vi "UHR-Fleezers Control (host) - 11.9b.vi"() -> ()   [LabVIEW 2014] (continued)
  # "Fl. Up"
  # "Bead sep"
  # "Trap Display:"
  # "APD Display:"
  # "Trap Manipulation"
  # "Data Saving"
  # "DAQ"
  # "Bead Calibration"
  # "Tether screen"
  # "Bottom Pump (#1)"
  # "Central Sample Channels"
  # "Top Pump (#3)"
  # "Rate param is ul/h\nVolume param is ul"
  # "Chemyx Pump 2"
  # "Units: \n1 = ml/m\n2 = ml/h\n3 = ul/m\n4 = ul/h"
  # "X"
  # "Y"
  # "Oscillate Set 1 freq. (debugging)"
  # "BD 1"
  # "BD 2"
  # "AOD Raster Scan"
  # "Approx. trap separations"
  # "X"
  # "Y"
  # "FPGA\nreading"
  # "DMA\ntransfer"
  # "APD Gates"
  # "APD 2"
  # "APD 1"
  # "X"
  # "2D"
  # "Y"
  # "1D"
  # "Green Laser Interlacing"
  # "Green FB Measurement"
  # "Digital Gate"
  # "Current Analog Control"
  # "Total AI Rates (NOT rates/trap)"
  # "(Samples/trap x Trap Sets)"
  # "(Samples/channel x\n8 if averaging (8 channels)\n4 if no averaging)"
  # "Trap 1"
  # "Trap 2"
  # "Flour./Trap 3"
  # "External Video Window"
  # "MCL Position Debugging"
  # "Temporary Control Storage\n(these used to be somewhere else, still want to keep them)"
  # "Y"
  # "X"
  # "Trap Position Difference Limits"
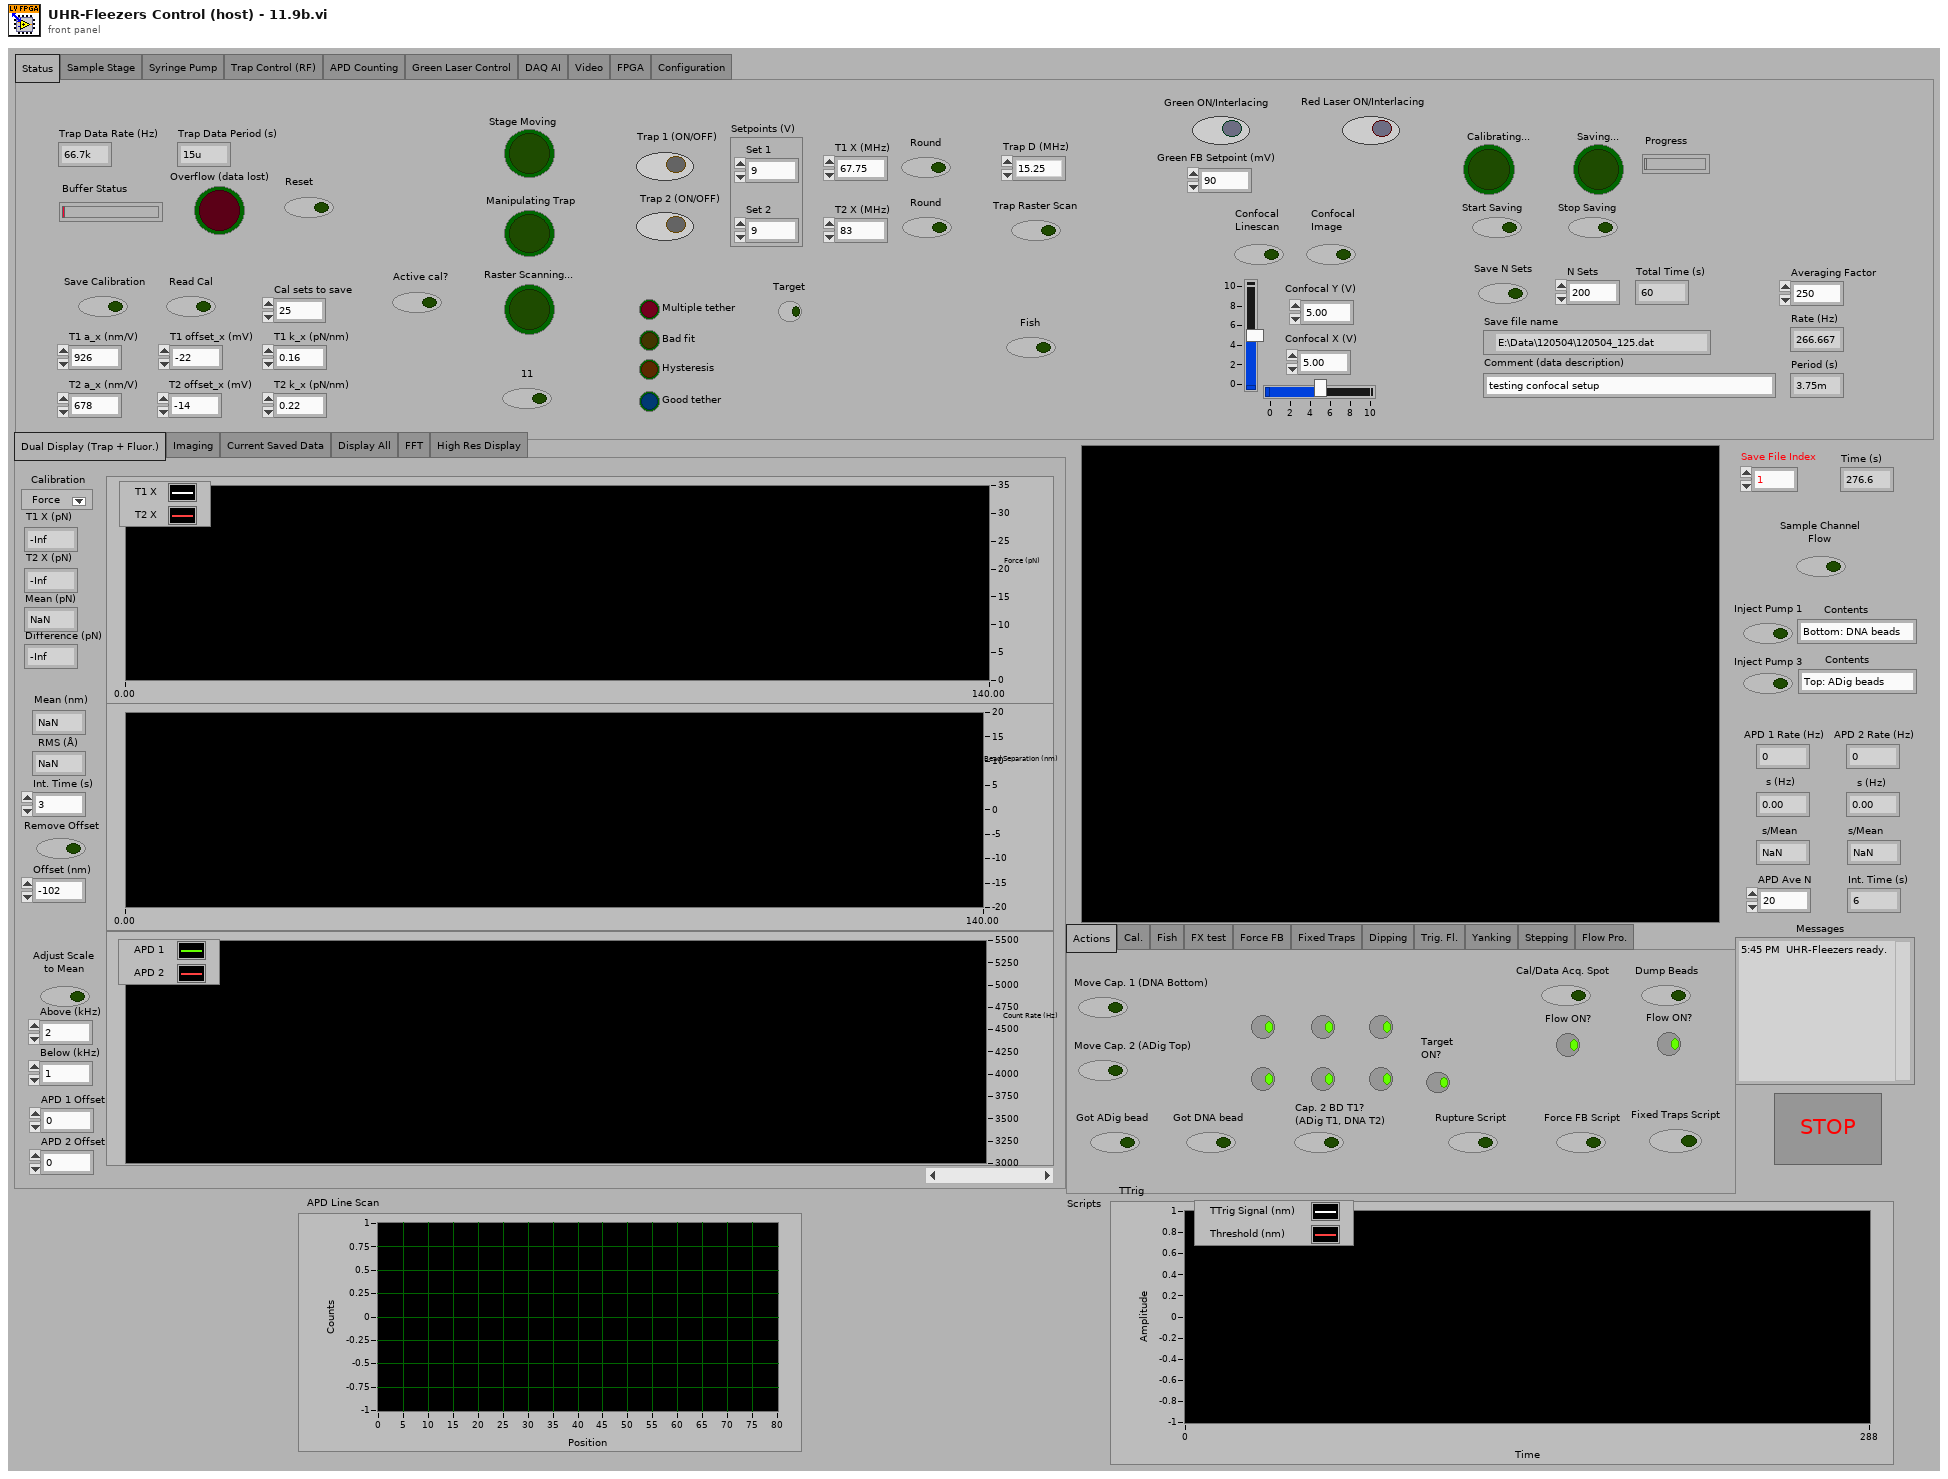
[diagram p1: front panel]
types:
  T1 = enum32{"Actions", "Cal.", "Fish", "FX test", "Force FB", "Fixed Traps", "Dipping", "Trig. Fl.", "Yanking", "Stepping", "Flow Pro."}
  T2 = typedef "IMAQ Image.ctl" = refnum<image>
  T3 = enum32{"Dual Display (Trap + Fluor.)", "Imaging", "Current Saved Data", "Display All", "FFT", "High Res Display"}
  T4 = enum32{"Status", "Sample Stage", "Syringe Pump", "Trap Control (RF)", "APD Counting", "Green Laser Control", "DAQ AI", "Video", "FPGA", "Configuration"}
  T5 = cluster{"Pump 1":cluster{"Diameter (mm)":dbl, "Units":dbl, "Volume":dbl, "Rate":dbl}, "Pump 2":cluster{"Diameter (mm)":dbl, "Units":dbl, "Volume":dbl, "Rate":dbl}, "Pump 3":cluster{"Diameter (mm)":dbl, "Units":dbl, "Volume":dbl, "Rate":dbl}}
  T6 = enum32{"IR Laser Interlacing (Direct RF Board Control Method)", "AOD Raster Scan", "Feedback on Trap Intensity", "Feedback on Trap Position"}
  T7 = typedef "LVPoint32TypeDef.ctl" = cluster{"Horizontal":i32, "Vertical":i32}
  T8 = cluster{"Scan Range AOD (nm) 2":dbl, "Step Size AOD (nm) 2":dbl, "Scan Speed AOD (nm/s) 2":dbl, "Number of scans (AOD) 2":u16, "Label":string}[]
  T9 = cluster{"Set 1":cluster{"proportional gain (Kc)":i16, "integral gain (Kc*Ts/Ti)":i16, "derivative gain (Kc*Td/Ts)":i16}, "Set 2":cluster{"proportional gain (Kc)":i16, "integral gain (Kc*Ts/Ti)":i16, "derivative gain (Kc*Td/Ts)":i16}}
  T10 = cluster{"Trap 1":fxp<+/-,16,1>, "Trap 2":fxp<+/-,16,1>}
  T11 = cluster{"proportional gain (Kc)":fxp<+/-,16,8>, "integral gain (Kc*Ts/Ti)":fxp<+/-,16,8>, "derivative gain (Kc*Td/Ts)":fxp<+/-,16,8>}
  T12 = cluster{"output high":fxp<+/-,64,32>, "output low":fxp<+/-,64,32>}
  T13 = cluster{"Set 1":fxp<+/-,16,1>, "Set 2":fxp<+/-,16,1>}
  T14 = cluster{"proportional gain (Kc)":i16, "integral gain (Kc*Ts/Ti)":i16, "derivative gain (Kc*Td/Ts)":i16}
  T15 = cluster{"Set 1":bool, "Set 2":bool, "Set 3":bool}
  T16 = typedef "LVMinMaxIncTypeDef.ctl" = cluster{"Minimum":dbl, "Maximum":dbl, "Increment":dbl}
  T17 = typedef "Image Type" = u32
  T18 = typedef "nirio_resource_hc.ctl" = tag
  T19 = typedef "openfpgaref.8.6.ctl" = refnum<k20>
  T20 = cluster{"New Image":T2, "New Image":T2, "New Image":T2, "New Image":T2}
  T21 = typedef "XDNodeRunTimeDep.lvlib/timing_clust.ctl" = cluster{"Expected End [f-1]":u64, "Actual End [f-1]":u64, "Finished Late? [f-1]":bool, "Expected End [i-1]":u64, "Actual End [i-1]":u64, "Finished Late? [i-1]":bool, "Expected Start [i]":u64, "Actual Start [i]":u64, "Expected Start [f]":u64, "Actual Start [f]":u64, "Source Name":string, "Structure Name":string, "Period":i64, "Deadline":i64, "Offset":i64, "Start":i64, "Priority":i32, "Timeout":i32, "Mode":T22, "Wakeup Reason":T23, "Error":errorcluster, "Source Type":string, "Secondary Source Type":string, "Global End Time":u64, "Global Start Time":u64, "Frame Duration":u64, "Iteration Duration":u64, "Assigned CPU":i32, "I/O Scan Engine Mode":u32}
  T22 = typedef "XDNodeRunTimeDep.lvlib/nitl_modes.ctl" = enum32{"No Change", "Process missed periods, maintain original phase", "Discard missed periods, maintain original phase", "Process missed periods, ignore original phase", "Discard missed periods, ignore original phase"}
  T23 = typedef "XDNodeRunTimeDep.lvlib/wakeup.ctl" = enum32{"Normal", "Aborted", "Asynchronous wakeup", "Timing source error", "Timed loop error", "Timeout"}
  T24 = enum16{"big-endian, network order", "native, host order", "little-endian"}
  T25 = enum16{"open", "replace", "create", "open or create", "replace or create", "replace or create with confirmation"}
  T26 = cluster{"Scan Range AOD (nm) 2":dbl, "Step Size AOD (nm) 2":dbl, "Scan Speed AOD (nm/s) 2":dbl, "Number of scans (AOD) 2":u16, "Label":string}
  T27 = cluster{"[0]":dbl, "[1]":dbl, "[2]":dbl, "[3]":dbl, "[4]":dbl, "[5]":dbl}
  T28 = cluster{"Diameter (mm)":dbl, "Units":dbl, "Volume":dbl, "Rate":dbl}
  T29 = enum16{"Actions", "Cal.", "Fish", "FX test", "Force FB", "Fixed Traps", "Dipping", "Trig. Fl.", "Yanking", "Stepping", "Flow Pro."}
  T30 = cluster{"Left":i32, "Top":i32, "Width":u32, "Height":u32}
  T31 = cluster{cluster{"Left":i32, "Top":i32, "Width":u32, "Height":u32}}[]
  T32 = enum32{"setting", "request", "request control", "info", "statistics", "system settings", "I/O sub system", "HRT control", "camera descriptions", "device specific data", "event sub system settings", "event sub system results", "image memory manager"}
  T33 = typedef "AviRefnum.ctl" = refnum<k1>
  T34 = typedef "imagedata.ctl" = cluster{"image type":i32, "image depth":i32, "image":u8[], "mask":u8[], "colors":u32[], "Rectangle":cluster{"left":i16, "top":i16, "right":i16, "bottom":i16}}
  T35 = enum32{"Normal Display", "Dual Display (APD)", "FFT", "High Res Display"}
  T36 = cluster{"Origin Pixel":cluster{"X":sgl, "Y":sgl}, "Angle Relative to Horizontal (deg)":sgl, "Axis Reference":u32}
  T37 = typedef "Simple Grid Descriptor" = cluster{"X Step":sgl, "Y Step":sgl, "Unit":T38}
  T38 = typedef "Image Unit" = enum32{"Undefined", "Angström", "Micrometer", "Millimeter", "Centimeter", "Meter", "Kilometer", "Microinch", "Inch", "Feet", "Nautical miles", "Standard miles", "Steps"}
  T39 = cluster{"averaging mode":u16, "weighting mode":u16, "number of averages":u32}
  T40 = cluster{"dB On (F)":bool, "unwrap phase (F)":bool, "convert to degree (F)":bool}
  T41 = cluster{string, string, string, string, string, string, string, string}
  T42 = cluster{string, string, string, string, string, string, string, string, string, string, string, string}
  T43 = cluster{string, string, string, string, string, string, string, string, string, string, string, string, string}
  T44 = cluster{string, string, string, string, string, string, string, string, string, string, string, string, string, string}
  T45 = cluster{"BD 1 Frequency 1 (MHz)":dbl, "BD 1 Frequency 2 (MHz)":dbl}
  T46 = cluster{"f0":dbl, "df":dbl, "magnitude":dbl[]}[][]
  T47 = cluster{"Green FB Ch 0":i16, "Green FB Ch 1":i16, "Green FB Ch 2":i16}
  T48 = cluster{"Green FB Ch 0":dbl, "Green FB Ch 1":dbl, "Green FB Ch 2":dbl}
diagram:
  w17 = 0.0 ("Total Volume\nFlowed P1 (uL)")
  w29 = u16 20 items=["1.0"=10, "1.5"=15, "2.0"=20] ("stop bits (10: 1 bit)")
  w32 = u16 20 items=["1.0"=10, "1.5"=15, "2.0"=20] ("stop bits (10: 1 bit)")
  w89 = u16 20 items=["1.0"=10, "1.5"=15, "2.0"=20] ("stop bits (10: 1 bit)")
  w96 = T17 2 items=["Grayscale (U8)", "Grayscale (I16)", "Grayscale (SGL)", "Complex (CSG)", "RGB (U32)", "HSL (U32)", "RGB (U64)", "Grayscale (U16)"] ("Image Type")
  w158 = cluster{"output high":i16, "output low":i16} {"output high"=3000, "output low"=0} ("FB output range 1")
  w229 = 10.0 ("y")
  w228 = 32767.0 ("y")
  w244 = 6.0  # clock mult.
  w245 = 49152000.0  # TCXO frequ.
  # "Bottom 1 Harvard"
  # "Top 3 Harvard"
  # "Center Harvard"
  # "Bottom 1 Harvard"
  # "Top 3 Harvard"
  # "Center Harvard"
  n1 = Build Array("DIO count 1 (ticks)", "DIO count 2 (ticks)", "DIO count 3 (ticks)") -> (w145:u32[])
  n2 = local read "AO1"() -> (w223:dbl)
  n3 = local read "AO2"() -> (w222:dbl)
  n4 = local read "Scan Increment (MHz)"() -> (w240:dbl)
  n5 = local read "Continuous MCL Scanning"() -> (w210:bool)
  n6 = local read "Fast Scan Dir"() -> (w209:bool)
  n7 = local read "Number of scans (MCL)"() -> (w211:u64)
  n8 = property on="AI Count (ticks)" class="DigNum (strict)"("Val(Sgnl)"="AI Count (ticks)") -> ()  [unwired: 2 in, 2 out]
  n9 = Multiply(x=w223, y=w228) -> (x*y=w225:dbl)
  n10 = Multiply(x=w222, y=w228) -> (x*y=w227:dbl)
  n11 = Divide(x=w225, y=w229) -> (x/y=w224:dbl)
  n12 = Divide(x=w227, y=w229) -> (x/y=w226:dbl)
  n13 = To Word Integer(number=w224) -> (16bit integer=w221:i16)
  n14 = To Word Integer(number=w226) -> (16bit integer=w220:i16)
  n15 = Not(x=w209) -> (.not. x?=w204:bool)
  n16 = local read "Cycles/step (MCL)"() -> (w212:u64)
  n17 = Multiply(x=w240, y=1000.0) -> (x*y=w247:dbl)
  n18 = local read "Scan steps (MCL)"() -> (w213:u64)
  n19 = local write "Trap Pos FIFO Timeout"(u16 0 ("Trap Pos FIFO Timeout")) -> ()
  n20 = local read "Desired Scan Incr (V)"() -> (w215:dbl)
  n21 = Scale By Power Of 2(n=48, x=w247) -> (x*2^n=w248:dbl)
  n22 = Multiply(x=w245, y=w244) -> (x*y=w243:dbl)
  n23 = Divide(x=w248, y=w243) -> (x/y=w242:dbl)
  n24 = local read "Setpoints (V)"() -> (w259:cluster{"Set 1":dbl, "Set 2":dbl})
  n25 = To Quad Integer(1:w242) -> (0:w239:i64)
  n26 = Divide(x=40000000.0, y="AI Count (ticks)") -> (x/y=w200:dbl)
  n27 = Multiply(x=w215, y=32767.0) -> (x*y=w217:dbl)
  n28 = local read "Number Interlace Sets"() -> (w138:u8)
  n29 = Split 1D Array(array=w145, index=w138) -> (first subarray=w147:u32[])  [unwired: 1 out]
  n30 = Add Array Elements(numeric array=w147) -> (sum=w146:u32)
  n31 = local read "# Samples/channel"() -> (w232:u32)
  n32 = local read "Number of F/B Scans (AOD)"() -> (w233:u16)
  n33 = local read "Not-Interlacing Set"() -> (w137:enum32{"Set 1", "Set 2", "Set 3"})
  n34 = To Unsigned Byte Integer(number=w137) -> (unsigned 8bit integer=w143:u8)
  n35 = Index Array(array=w145, index=w143) -> (element=w144:u32)
  n36 = local read "Feedback On/Off"() -> (w262:cluster{"Set 1":bool, "Set 2":bool})
  n37 = local read "PID Gains"() -> (w254:T9)
  n38 = local read "Scan steps (AOD)"() -> (w238:u64)
  n39 = local read "All FB On/Off"() -> (w263:bool)
  n40 = local read "Cycles/step (AOD)"() -> (w237:u64)
  n41 = local write "AI rate (Hz)"(w200) -> ()
  n42 = Divide(x=w217, y=10.0) -> (x/y=w216:dbl)
  n43 = Multiply(x=w238, y=w237) -> (x*y=w236:u64)
  n44 = Multiply(x=3276.7, y=w259) -> (x*y=w258:cluster{"Set 1":dbl, "Set 2":dbl})
  n45 = To Word Integer(number=w216) -> (16bit integer=w214:i16)
  n46 = xnode "Open FPGA VI Reference"("resource name"=T18 "RIO1") -> ("FPGA VI Reference Out"=w15:T19, "error out"=w13:errorcluster)  [unwired: 1 in]
  n47 = Multiply(x=w236, y=u64 2) -> (x*y=w234:u64)
  n48 = local read "Sets to FIFO (Traps)"() -> (w266:T15)
  n49 = Divide(x=w200, y="FPGA Ave.") -> (x/y=w201:dbl)
  n50 = To Word Integer(number=w258) -> (16bit integer=w257:cluster{"Set 1":i16, "Set 2":i16})
  n51 = Unbundle By Name(w254) -> ("Set 1"=w253:T14, "Set 2"=w252:T14)
  n52 = Multiply(x=w234, y=w233) -> (x*y=w231:u64)
  n53 = local write "Ave. Rate (Hz)"(w201) -> ()
  n54 = Divide(x=w231, y=w232) -> (x/y=w230:dbl)
  n55 = Unbundle By Name(w257) -> ("Set 1"=w256:i16, "Set 2"=w255:i16)
  n56 = local read "2D or 1D Scan"() -> (w159:bool)
  n57 = local write "Data points/scans"(w231) -> ()
  n58 = local read "Scan BD"() -> (w249:bool)
  n59 = And(x=w262, y=w263) -> (x .and. y?=w261:cluster{"Set 1":bool, "Set 2":bool})
  n60 = local write "Data points/scan (f/b)"(w234) -> ()
  n61 = Reciprocal(x=w201) -> (1/x=w202:dbl)
  n62 = local read "N Acq Sets (Traps + Fl.)"() -> (w193:i16)
  n63 = local write "N sets should be saved"(w230) -> ()
  n64 = xnode "Invoke Method"("FPGA VI Reference In"=w15, "error in"=w13) -> ("FPGA VI Reference Out"=w157:T19, "error out"=w167:errorcluster)
  n65 = Unbundle By Name(w261) -> ("Set 1"=w265:bool, "Set 2"=w264:bool)
  n66 = local read "Interlace"() -> (w139:bool)
  n67 = Select(t=w146, s=w139, f=w144) -> (s? t:f=w136:u32)
  n68 = local write "Update Count (MCL)"(w136) -> ()
  n69 = local write "Total Counts (ticks)"(w136) -> ()
  n70 = local write "Ave. Period (s)"(w202) -> ()
  n71 = property on="2D or 1D Scan" class="Bool (strict)"("Val(Sgnl)"=w159) -> ()  [unwired: 2 in, 2 out]
  n72 = local read "GI Frequency, OFF count"() -> (w61:u32)
  n73 = local read "GI Frequency, ON count"() -> (w52:u32)
  n74 = local read "APD Gate OFF Count"() -> (w58:u32)
  n75 = local read "APD Gate ON Count"() -> (w54:u32)
  n76 = xnode "Read/Write Control"("FPGA VI Reference In"=w156, "error in"=w167, "ai count"="AI Count (ticks)", "Interlace ON/OFF"=w139, "Number Interlace Cycles"=w138, "AI1 Sets to FIFO"=w266, "FB On/Off Set 1"=w265, "FB On/Off Set 2"=w264, "Interlace Off Parameters"=w137, "FB Setpoint Set 1"=w256, "FB Setpoint Set 2"=w255, "FB Gains Set 1"=w253, "FB Gains Set 2"=w252, "FB output range 1"=w158, "FB output range 2"=w158, "Cycles per step"=w237, "Scan BD"=w249, "Number of scans"=w233, "Scan steps"=w238, "Scan freq.  increment"=w239, "AO1"=w221, "AO2"=w220, "Scan freq.  increment (MCL)"=w214, "Scan steps (MCL)"=w213, "Cycles per step (MCL)"=w212, "Number of scans (MCL)"=w211, "MCL count"=w136, "Cont. Scan (MCL)"=w210, "MCL Scan Axis"=w204, "1D or 2D Scan?"=w159, "N of AI1 Int Acq Sets"=w193, "Freq or Amp switch first"="Freq or Amp switch first", "Freq switch delay"="Freq switch delay", "Amp switch delay"="Amp switch delay", "Swap F1 and F2"="Swap F1 and F2", "APD to FIFO"=FALSE, "DIO count 1 (ticks)"="DIO count 1 (ticks)", "DIO count 2 (ticks)"="DIO count 2 (ticks)", "DIO count 3 (ticks)"="DIO count 3 (ticks)") -> ("FPGA VI Reference Out"=w65:T19, "error out"=w63:errorcluster)  [unwired: 1 in]
  n77 = local read "On one out of X cycles"() -> (w60:u32)
  n78 = local read "APD Integration Time (s)"() -> (w44:dbl)
  n79 = local read "DMA Update Period (s)"() -> (w43:dbl)
  n80 = Add(x=w54, y=w58) -> (x+y=w56:u32)
  n81 = Add(x=w52, y=w61) -> (x+y=w59:u32)
  n82 = local read "Green ON/Interlacing"() -> (w134:bool)
  n83 = local read "Green laser mode"() -> (w135:enum32{"Laser ON", "Laser OFF", "Interlace"})
  n84 = Multiply(x=w56, y=w60) -> (x*y=w57:u32)
  n85 = Multiply(x=w60, y=w59) -> (x*y=w51:u32)
  n86 = Reciprocal(x=w44) -> (1/x=w41:dbl)
  n87 = Multiply(x=w44, y=40000000.0) -> (x*y=w40:dbl)
  n88 = Divide(x=w43, y=w44) -> (x/y=w46:dbl)
  n89 = Multiply(x="Current When FB OFF (%)", y=655.35) -> (x*y=w122:dbl)
  n90 = local read "Invert APD Gate"() -> (w50:bool)
  n91 = Multiply(x="Green FB Setpoint (mV)", y=3.2767) -> (x*y=w119:dbl)
  n92 = local read "APD Gate"() -> (w49:enum32{"ON", "OFF", "Interlace"})
  n93 = Subtract(x=w57, y=w54) -> (x-y=w55:u32)
  n94 = local write "Green FB Count"(w51) -> ()
  n95 = local write "APD Acq Rate (Hz)"(w41) -> ()
  n96 = To Unsigned Long Integer(number=w40) -> (unsigned 32bit integer=w38:u32)
  n97 = Multiply(x=2.0, y=w46) -> (x*y=w45:dbl)
  n98 = local read "Invert GI"() -> (w131:bool)
  n99 = To Unsigned Word Integer(number=w122) -> (unsigned 16bit integer=w120:u16)
  n100 = Subtract(x=w51, y=w52) -> (x-y=w53:u32)
  n101 = local write "APD Samples/FIFO Acq."(w46) -> ()
  n102 = To Word Integer(number=w119) -> (16bit integer=w117:i16)
  n103 = local write "APD Elements/DMA read"(w45) -> ()
  n104 = case shown="False" w134 {
    tunnel: w135 -> [_ w291]
    tunnel: [enum32{"Laser ON", "Laser OFF", "Interlace"}."Laser OFF" ("Green laser mode") w291] -> w130
    frame False {
    }
    frame True {
    }
  }
  n105 = local write "APD Int. Count"(w38) -> ()
  n106 = Multiply(x="Red current when FB OFF (%)", y=655.35) -> (x*y=w2:dbl)
  n107 = local read "Trap Pos. AI1 X Pre-scale"() -> (w75:u16)
  n108 = local read "Trap Pos FB Monitor\nT1 or T2"() -> (w82:bool)
  n109 = To Unsigned Word Integer(number=w2) -> (unsigned 16bit integer=w1:u16)
  n110 = local read "Trap Pos FB Int Count"() -> (w69:u16)
  n111 = local read "APD 1 AO Mult."() -> (w48:i16)
  n112 = local read "Trap Pos FB Negate Action"() -> (w81:bool)
  n113 = local read "APD 2 AO Mult."() -> (w47:i16)
  n114 = local read "Trap Pos. FB Offset Factor"() -> (w80:i64)
  n115 = local read "Trap Pos. FB Mult Factor"() -> (w79:i64)
  n116 = local read "Differential FB?"() -> (w35:bool)
  n117 = local read "Neg. TTrig FPGA"() -> (w37:bool)
  n118 = local read "Trap Pos. FB Gains"() -> (w77:T11)
  n119 = local read "Trap Pos. FB Range"() -> (w78:T12)
  n120 = xnode "Read/Write Control"("FPGA VI Reference In"=w65, "error in"=w63, "Invert APD Gate"=w50, "APD Gate ON Count"=w54, "APD Gate OFF Count"=w55, "APD Acq Rate Count"=w38, "APD Gate Operating Mode"=w49, "APD 1 AO scale factor"=w48, "APD 2 AO scale factor"=w47, "Green interlace ON count"=w52, "Green interlace OFF count"=w53, "Green interlace ON count 2"=w52, "Green interlace OFF count 2"=w53, "Green FB Count"=w51) -> ("FPGA VI Reference Out"=w64:T19, "error out"=w62:errorcluster)
  n121 = xnode "Read/Write Control"("FPGA VI Reference In"=w64, "error in"=w62, "Invert GI 2"=w131, "Operating Mode 2"=w130, "Green FB Gains"="Green FB Gains", "Green FB Setpoint"=w117, "Green FB On/Off"="Green FB On/Off", "Current Out"=w120, "Green int current ON count adj"="Green int current ON count adj", "Operating Mode"=w130, "Invert GI"=w131, "Trap Pos FB Monitor T1 or T2"=w82, "Trap Pos FB Negate Action"=w81, "Trap Pos. FB Offset Factor"=w80, "Trap Pos. FB Mult Factor"=w79, "Trap Pos. FB Range"=w78, "Trap Pos. FB Gains"=w77, "Force feedback"=FALSE, "AI1 X Scale"=w75, "Trap Pos to FIFO"=TRUE, "Trap Pos FB Int Count"=w69, "TTrig Negate Pos"=w37, "FB Trig Integrate"="FB Trig Integrate", "Diff FB Measurement?"=w35, "Negate Diff?"="Negate Diff?", "RI Current Out"=w1) -> ("FPGA VI Reference Out"=w132:T19, "error out"=w133:errorcluster)
  n122 = xnode "Invoke Method"("FPGA VI Reference In"=w132, "error in"=w133, "Requested Depth"="Trap AI FIFO Depth") -> ("FPGA VI Reference Out"=w85:T19, "error out"=w84:errorcluster)  [unwired: 1 out]
  n123 = xnode "Invoke Method"("FPGA VI Reference In"=w85, "error in"=w84, "Requested Depth"="Trap Position FIFO Depth") -> ("FPGA VI Reference Out"=w71:T19, "error out"=w70:errorcluster)  [unwired: 1 out]
  n124 = flat-sequence {
    tunnel: w157 -> [w296]
    tunnel: [w296] -> w156
    tunnel: [w295] -> w155
    tunnel: [w294] -> w154
    tunnel: [w292] -> w152
    tunnel: [w293] -> w153
    frame #0 {
      w293 = T16 {"Minimum"=0.0, "Maximum"=40.0, "Increment"=1.0} ("Min Max Inc")
      w292 = T16 {"Minimum"=0.0, "Maximum"=50.0, "Increment"=1.0} ("Data Entry Limits")
      w295 = T16 {"Minimum"=60.0, "Maximum"=90.0, "Increment"=1.0} ("Min Max Inc")
      w294 = T16 {"Minimum"=0.0, "Maximum"=50.0, "Increment"=1.0} ("Data Entry Limits")
      n125 = property on="BD 2 Frequency 1 (MHz)" class="DigNum (strict)"("Data Range"=w293) -> ()  [unwired: 2 in, 2 out]
      n126 = property on="BD 2 Frequency 3 (MHz)" class="DigNum (strict)"("Data Range"=w293) -> ()  [unwired: 2 in, 2 out]
      n127 = property on="BD 2 Frequency 2 (MHz)" class="DigNum (strict)"("Data Range"=w293) -> ()  [unwired: 2 in, 2 out]
      n128 = property on="BD 1 Frequency 1 (MHz)" class="DigNum (strict)"("Data Range"=w295) -> ()  [unwired: 2 in, 2 out]
      n129 = property on="BD 1 Frequency 2 (MHz)" class="DigNum (strict)"("Data Range"=w295) -> ()  [unwired: 2 in, 2 out]
      n130 = property on="BD 1 Frequency 3 (MHz)" class="DigNum (strict)"("Data Range"=w295) -> ()  [unwired: 2 in, 2 out]
      n131 = property on="BD 2 Amplitude 1 (%)" class="DigNum (strict)"("Data Range"=w292) -> ()  [unwired: 2 in, 2 out]
      n132 = property on="BD 2 Amplitude 2 (%)" class="DigNum (strict)"("Data Range"=w292) -> ()  [unwired: 2 in, 2 out]
      n133 = property on="BD 2 Amplitude 3 (%)" class="DigNum (strict)"("Data Range"=w292) -> ()  [unwired: 2 in, 2 out]
      n134 = property on="BD 1 Amplitude 3 (%)" class="DigNum (strict)"("Data Range"=w294) -> ()  [unwired: 2 in, 2 out]
      n135 = property on="BD 1 Amplitude 2 (%)" class="DigNum (strict)"("Data Range"=w294) -> ()  [unwired: 2 in, 2 out]
      n136 = property on="BD 1 Amplitude 1 (%)" class="DigNum (strict)"("Data Range"=w294) -> ()  [unwired: 2 in, 2 out]
      "X RF Frequency Limits (MHz)" <- w295
      "X RF Amplitude Limits (%)" <- w294
      "Y RF Amplitude Limits (%)" <- w292
      "Y RF Frequency Limits (MHz)" <- w293
    }
  }
  n137 = xnode "Invoke Method"("FPGA VI Reference In"=w71, "error in"=w70) -> ("FPGA VI Reference Out"=w166:T19, "error out"=w165:errorcluster)  [unwired: 1 in]
  n138 = flat-sequence "Initial FPGA Loop Relative Phase Adjustment" {
    tunnel: "Initial Phase Adjustment (APD 2 Gate)" -> [w299]
    tunnel: "Initial Phase Adjustment (GI) 2" -> [w300]
    tunnel: "Initial Phase Adj. (MCL)" -> [w298]
    tunnel: w165 -> [w301]
    tunnel: w166 -> [w302]
    tunnel: "Initial Phase Adjustment (GI)" -> [w303]
    tunnel: "Initial Phase Adjustment (AI1)" -> [w304]
    tunnel: [w304] -> w12
    tunnel: [w303] -> w11
    tunnel: [w302] -> w10
    tunnel: [w301] -> w9
    tunnel: [w298] -> w8
    tunnel: [w300] -> w7
    tunnel: [w299] -> w6
    tunnel: [w316] -> w175
    tunnel: [w310] -> w171
    tunnel: "Initial Phase Adjustment (APD Acq)" -> [w309]
    tunnel: "Initial Phase Adjustment (APD 1 Gate)" -> [w308]
    tunnel: "Initial Phase Adjustment (Green FB)" -> [w307]
    tunnel: w12 -> [w315]
    tunnel: w11 -> [w314]
    tunnel: w10 -> [w313]
    tunnel: w9 -> [w312]
    tunnel: w8 -> [w311]
    tunnel: w7 -> [w306]
    tunnel: w6 -> [w305]
    tunnel: w175 -> [w318]
    tunnel: [w319] -> w172
    tunnel: w171 -> [w319]
    tunnel: [w318] -> w170
    tunnel: w172 -> [w322]
    tunnel: w170 -> [w321]
    tunnel: [w324] -> w169
    tunnel: [w323] -> w168
    tunnel: [w326] -> w173
    tunnel: [w327] -> w174
    tunnel: w169 -> [w327]
    tunnel: w168 -> [w326]
    frame #0 {
      n139 = Wait (ms)(milliseconds to wait=u32 100) -> ()  [unwired: 1 out]
    }
    frame #1 {
      n140 = xnode "Read/Write Control"("FPGA VI Reference In"=w313, "error in"=w312, "Phase count adjustment"=w315, "Phase count adjustment (GI)"=w314, "Phase count adjustment (MCL)"=w311, "Phase Count Adjustment (APD Acq)"=w309, "Phase count adjustment (APD 1 Gate)"=w308, "Phase count adjustment (APD 2 Gate)"=w305, "Phase count adjustment (Green FB)"=w307, "Phase count adjustment (GI) 2"=w306) -> ("FPGA VI Reference Out"=w310:T19, "error out"=w316:errorcluster)
    }
    frame #2 {
      n141 = Wait (ms)(milliseconds to wait=u32 100) -> ()  [unwired: 1 out]
    }
    frame #3 {
      w320 = TRUE
      n142 = xnode "Read/Write Control"("FPGA VI Reference In"=w322, "error in"=w321, "+ phase"=w320, "+ phase (GI)"=w320, "+ phase (MCL)"=w320, "+ phase (APD Acq)"=w320, "+ phase (APD 1 Gate)"=w320, "+ phase (APD 2 Gate)"=w320, "+ phase (Green FB)"=w320, "+ phase (GI) 2"=w320) -> ("FPGA VI Reference Out"=w323:T19, "error out"=w324:errorcluster)
    }
    frame #4 {
      n143 = Wait (ms)(milliseconds to wait=u32 100) -> ()  [unwired: 1 out]
    }
  }
  n144 = local read "Phase adj. (Green FB)"() -> (w148:i16)
  n145 = local read "Phase adj. (GI) 2"() -> (w123:i16)
  n146 = local read "Phase adjust (MCL)"() -> (w205:i16)
  n147 = local read "Phase adj. (AI1)"() -> (w207:i16)
  n148 = local read "Phase adj. (GI)"() -> (w206:i16)
  n149 = xnode "Read/Write Control"("FPGA VI Reference In"=w173, "error in"=w174, "Phase count adjustment"=w207, "Phase count adjustment (GI)"=w206, "Phase count adjustment (MCL)"=w205, "Phase Count Adjustment (APD Acq)"="Phase Adj. (APD Acq)", "Phase count adjustment (APD 1 Gate)"="Phase Adj. (APD 1 Gate)", "Phase count adjustment (APD 2 Gate)"="Phase Adj. (APD 2 Gate)", "Phase count adjustment (Green FB)"=w148, "Phase count adjustment (GI) 2"=w123) -> ("FPGA VI Reference Out"=w14:T19, "error out"=w182:errorcluster)
  n150 = call "Initialize RF boards - interlace 3.vi"("error in"=w182, "FPGA VI Reference In"=w14) -> ("error out"=w180:errorcluster, "FPGA VI Reference Out"=w181:T19)
  n151 = call "set RF board frequency - interlace.vi"("Board 2 Frequency Limits"=w153, "Board 1 Frequency Limits"=w155, "error in"=w180, "FPGA VI Reference In"=w181, "Board 2 Frequency 3 (MHz)"="BD 2 Frequency 3 (MHz)", "Board 1 Frequency 3 (MHz)"="BD 1 Frequency 3 (MHz)", "Board 2 Frequency 2 (MHz)"="BD 2 Frequency 2 (MHz)", "Board 2 Frequency 1 (MHz)"="BD 2 Frequency 1 (MHz)", "Board 1 Frequency 2 (MHz)"="BD 1 Frequency 2 (MHz)", "Board 1 Frequency 1  (MHz)"="BD 1 Frequency 1 (MHz)") -> ("error out"=w281:errorcluster, "FPGA VI Reference Out"=w282:T19)
  n152 = call "set RF board amplitude - interlace.vi"("Board 2 Amplitude Limits"=w152, "Board 1 Amplitude Limits"=w154, "error in"=w281, "FPGA VI Reference In"=w282, "Board 2 Amplitude 3 (%)"="BD 2 Amplitude 3 (%)", "Board 1 Amplitude 3 (%)"="BD 1 Amplitude 3 (%)", "Board 2 Amplitude 2 (%)"="BD 2 Amplitude 2 (%)", "Board 2 Amplitude 1 (%)"="BD 2 Amplitude 1 (%)", "Board 1 Amplitude 2 (%)"="BD 1 Amplitude 2 (%)", "Board 1 Amplitude 1 (%)"="BD 1 Amplitude 1 (%)") -> ("error out"=w269:errorcluster, "FPGA VI Reference Out"=w270:T19)
  n153 = flat-sequence {
    tunnel: w270 -> [w337]
    tunnel: w269 -> [w336]
    tunnel: [w335] -> w274
    tunnel: [w334] -> w273
    tunnel: [w341] -> w272
    tunnel: w274 -> [w341]
    tunnel: [w340] -> w271
    tunnel: w273 -> [w340]
    tunnel: w272 -> [w350]
    tunnel: w271 -> [w349]
    tunnel: [w348] -> w23
    tunnel: [w347] -> w72
    frame #0 {
      w328 = FALSE ("Retract Pump 3")
      n154 = local read "Trap 1 (ON/OFF)"() -> (w329:bool)
      n155 = xnode "Read/Write Control"("FPGA VI Reference In"=w337, "error in"=w336, "Direct RF Box  Communication"=FALSE) -> ("FPGA VI Reference Out"=w335:T19, "error out"=w334:errorcluster)
      n156 = local write "Saving..."(FALSE ("Saving Data")) -> ()
      n157 = local write "Stop All"(FALSE ("Stop All")) -> ()
      n158 = local write "Retract Pump 1"(w328) -> ()
      n159 = local write "Retract Pump 3"(w328) -> ()
      n160 = local write "Index"(1.0 ("Index")) -> ()
      n161 = property on="Trap 1 ON" class="Bool (strict)"("Value"=w329) -> ()  [unwired: 2 in, 2 out]
      "Manipulating Trap" <- FALSE ("Manipulating Trap")
    }
    frame #1 {
      n162 = local read "Trap 2 (ON/OFF)"() -> (w339:bool)
      n163 = Wait (ms)(milliseconds to wait=u32 10) -> ()  [unwired: 1 out]
      n164 = property on="Trap 2 ON" class="Bool (strict)"("Val(Sgnl)"=w339) -> ()  [unwired: 2 in, 2 out]
    }
    frame #2 {
      n165 = local read "Scan Range (nm)"() -> (w343:dbl)
      n166 = xnode "Read/Write Control"("FPGA VI Reference In"=w350, "error in"=w349, "FPGA Controls  RF Box"=TRUE ("Direct RF Box  Communication")) -> ("FPGA VI Reference Out"=w348:T19, "error out"=w347:errorcluster)
      n167 = call "Update messages.vi"("Message to add"="UHR-Fleezers ready.", "Old message string"="") -> ("New message string"=w346:string)
      n168 = local write "Messages"(w346) -> ()
      n169 = property on="Scan Range (nm)" class="DigNum (strict)"("Val(Sgnl)"=w343) -> ()  [unwired: 2 in, 2 out]
    }
  }
  n170 = Subtract(x="BD 1 Frequency 1 (MHz)", y="BD 1 Frequency 2 (MHz)") -> (x-y=w192:dbl)
  n171 = Subtract(x="BD 2 Frequency 1 (MHz)", y="BD 2 Frequency 2 (MHz)") -> (x-y=w191:dbl)
  n172 = Square(x=w191) -> (x^2=w189:dbl)
  n173 = Square(x=w192) -> (x^2=w190:dbl)
  n174 = Add(x=w190, y=w189) -> (x+y=w188:dbl)
  n175 = Square Root(x=w188) -> (sqrt(x)=w187:dbl)
  n176 = local write "Trap D (MHz)"(w187) -> ()
  n177 = call "IMAQ Create"("Image Name"="APD 1 Image", "Image Type"=w96) -> ("New Image"=w95:T2)  [unwired: 3 in, 1 out]
  n178 = call "IMAQ Create"("Image Name"="APD 2 Image", "Image Type"=w96) -> ("New Image"=w94:T2)  [unwired: 3 in, 1 out]
  n179 = call "IMAQ Create"("Image Name"="Det. X Image", "Image Type"=w96) -> ("New Image"=w93:T2)  [unwired: 3 in, 1 out]
  n180 = call "IMAQ Create"("Image Name"="Det. Y Image", "Image Type"=w96) -> ("New Image"=w92:T2)  [unwired: 3 in, 1 out]
  n181 = Bundle("New Image"=w95, "New Image"=w94, "New Image"=w93, "New Image"=w92) -> (w91:T20)  [unwired: 1 in]
  n182 = call-poly "VISA Configure Serial Port"("VISA resource name"="Bottom  1 Harvard Syringe Pump Serial Port", "baud rate (9600)"=u32 115200, "stop bits (10: 1 bit)"=w29) -> ("VISA resource name out"=w25:refnum<visa-resource-name>, "error out"=w24:errorcluster)  [unwired: 4 in, 7 out]
  n183 = call-poly "VISA Configure Serial Port"("VISA resource name"="Top 3 Harvard Syringe Pump Serial Port", "baud rate (9600)"=u32 115200, "stop bits (10: 1 bit)"=w32) -> ("VISA resource name out"=w27:refnum<visa-resource-name>, "error out"=w26:errorcluster)  [unwired: 4 in, 7 out]
  n184 = call-poly "VISA Configure Serial Port"("VISA resource name"="Sample Chamber Stage Serial Port") -> ("VISA resource name out"=w105:refnum<visa-resource-name>, "error out"=w106:errorcluster)  [unwired: 5 in, 8 out]
  "Stage Control Serial Error" <- w106
  n185 = call-poly "VISA Configure Serial Port"("VISA resource name"="Center Harvard Syringe Pump Serial Port", "baud rate (9600)"=u32 115200, "stop bits (10: 1 bit)"=w89) -> ("VISA resource name out"=w86:refnum<visa-resource-name>, "error out"=w87:errorcluster)  [unwired: 4 in, 7 out]
  n186 = disable-structure shown="Disabled" {
    disable-tunnel: [w353 _] -> w251
    disable-tunnel: w23 -> [w352 _]
    frame Disabled {
      n187 = node-c288() -> (w355:T21)  [unwired: 4 out]
      n188 = timed-loop "Rough control of MCL mirror stage (debugging)" {
        tunnel: w352 -> [w358]
        tunnel: [w357] -> w353
        timing: w355 -> [_]
        timing-out: [_] -> w354
        stop <- w357 stop-if-true
        n189 = node-c288() -> ()  [unwired: 2 out]
        n190 = case shown="1" "MCL Mode" {
          tunnel: w358 -> [_ w361 w408]
          frame 0, Default {
          }
          frame 1 {
            n191 = node-c288() -> (w363:T21)  [unwired: 4 out]
            n192 = timed-loop "Oscillate MCL mirror" {
              timing: w363 -> [_]
              timing-out: [_] -> w362
              tunnel: w361 -> [w402]
              i -> [w401]
              stop <- w364 stop-if-true
              n193 = node-c288() -> (w400:i64)  [unwired: 1 out]
              n194 = Multiply(x="AO1", y=32767.0) -> (x*y=w396:dbl)
              n195 = Multiply(x="AO2", y=32767.0) -> (x*y=w391:dbl)
              n196 = Divide(x=w396, y=10.0) -> (x/y=w397:dbl)
              n197 = Divide(x=w391, y=10.0) -> (x/y=w392:dbl)
              n198 = To Word Integer(number=w397) -> (16bit integer=w389:i16)
              n199 = To Word Integer(number=w392) -> (16bit integer=w388:i16)
              n200 = Divide(x=w400, y=i64 1000) -> (x/y=w371:dbl)
              n201 = Multiply(x=w371, y=w401) -> (x*y=w382:dbl)
              n202 = Multiply(x="Osc. freq. (Hz) 2", y=6.283185307179586) -> (x*y=w383:dbl)
              n203 = Multiply(x=w383, y=w382) -> (x*y=w381:dbl)
              n204 = Sine(x=w381) -> (sin(x)=w380:dbl)
              n205 = Multiply(x=w380, y="Osc. amp. (V)") -> (x*y=w378:dbl)
              n206 = Add(x=w378, y="Osc. center (V)") -> (x+y=w376:dbl)
              n207 = Divide(x=w376, y=10.0) -> (x/y=w374:dbl)
              n208 = Multiply(x=w374, y=32767.0) -> (x*y=w369:dbl)
              n209 = Select(t=w369, s="Scan axis", f=w389) -> (s? t:f=w387:dbl)
              n210 = Select(t=w388, s="Scan axis", f=w369) -> (s? t:f=w386:dbl)
              n211 = local read "MCL Mode"() -> (w368:u16)
              n212 = Not Equal?(x=w368, y=u16 1) -> (x != y?=w365:bool)
              n213 = local read "Stop All"() -> (w366:bool)
              n214 = xnode "Read/Write Control"("FPGA VI Reference In"=w402, "AO1"=w387, "AO2"=w386) -> ()  [unwired: 1 in, 2 out]
              n215 = Compound Arithmetic op=OR(w366, w365) -> (w364:bool)
              n216 = node-c288() -> ()  [unwired: 2 out]
            }
            n217 = node-c288(w362) -> ()  [unwired: 1 out]
          }
          frame 2 {
            n218 = case shown="True" "Start Scan" {
              tunnel: w408 -> [_ w420]
              frame False {
              }
              frame True {
                n219 = Subtract(x="End (V)", y="Begin (V)") -> (x-y=w416:dbl)
                n220 = Decrement(x="N Points") -> (x-1=w415:dbl)
                n221 = Divide(x=w416, y=w415) -> (x/y=w413:dbl)
                n222 = for {
                  N: "N Points" -> [_]
                  tunnel: "Begin (V)" -> [w433]
                  tunnel: w420 -> [w425]
                  tunnel: [w424] -> w419 mode=indexing
                  tunnel: w413 -> [w423]
                  tunnel: [w421] -> w412 mode=indexing
                  i -> [w432]
                  n223 = Multiply(x=w423, y=w432) -> (x*y=w431:dbl)
                  n224 = Add(x=w433, y=w431) -> (x+y=w428:dbl)
                  n225 = local read "Scan axis"() -> (w422:bool)
                  n226 = local read "AO1"() -> (w430:dbl)
                  n227 = local read "AO2"() -> (w429:dbl)
                  n228 = Select(t=w428, s=w422, f=w430) -> (s? t:f=w427:dbl)
                  n229 = Select(t=w429, s=w422, f=w428) -> (s? t:f=w426:dbl)
                  n230 = flat-sequence {
                    tunnel: w427 -> [w437]
                    tunnel: w426 -> [w436]
                    tunnel: w425 -> [w434]
                    tunnel: [w447] -> w424
                    tunnel: [w446] -> w421
                    frame #0 {
                      w440 = 10.0 ("y")
                      w435 = 32767.0 ("y")
                      n231 = Multiply(x=w437, y=w435) -> (x*y=w443:dbl)
                      n232 = Multiply(x=w436, y=w435) -> (x*y=w441:dbl)
                      n233 = Divide(x=w443, y=w440) -> (x/y=w444:dbl)
                      n234 = Divide(x=w441, y=w440) -> (x/y=w442:dbl)
                      n235 = To Word Integer(number=w444) -> (16bit integer=w438:i16)
                      n236 = To Word Integer(number=w442) -> (16bit integer=w439:i16)
                      n237 = xnode "Read/Write Control"("FPGA VI Reference In"=w434, "AO1"=w438, "AO2"=w439) -> ()  [unwired: 1 in, 2 out]
                    }
                    frame #1 {
                      n238 = Wait (ms)(milliseconds to wait="DAQ Delay (ms)") -> ()  [unwired: 1 out]
                    }
                    frame #2 {
                      n239 = local read "Slow mean"() -> (w447:dbl)
                      n240 = local read "Sigma"() -> (w446:dbl)
                    }
                  }
                }
                n241 = Bundle("Begin (V)"="Begin (V)", w413, w419) -> (→"MCL Scan":cluster{"Begin (V)":dbl, dbl, dbl[]})  [unwired: 1 out]
                n242 = Bundle("Begin (V)"="Begin (V)", w413, w412) -> (→"MCL Scan 2":cluster{"Begin (V)":dbl, dbl, dbl[]})  [unwired: 1 out]
              }
            }
          }
        }
        n243 = local read "Stop All"() -> (w357:bool)
        n244 = node-c288() -> ()  [unwired: 2 out]
      }
      n245 = node-c288(w354) -> ()  [unwired: 1 out]
    }
    frame Enabled {
    }
  }
  n246 = node-c288(3 ("Processor")) -> (w111:T21)  [unwired: 3 out]
  n247 = timed-loop "Oscillate Trap/AOM (fishing, debugging)" {
    tunnel: w23 -> [w451]
    tunnel: [w450] -> w116
    timing: w111 -> [_]
    timing-out: [_] -> w110
    stop <- w450 stop-if-true
    n248 = node-c288() -> ()  [unwired: 2 out]
    n249 = event shown="[0] \"Oscillate Set 1\", \"Fish\": Value Change" {
      selector: _ -> [_ _ _]
      dyn-events: _ -> [_ _ _]
      timeout: _ -> [_ _ _]
      tunnel: w451 -> [w458 _ _]
      tunnel: [FALSE ("Stop All") _ w1143] -> w450
      event "Oscillate Set 1", "Fish": Value Change {
        n250 = event-data() -> ()  [unwired: 6 out]
        n251 = local read "Oscillate Set 1"() -> (w457:bool)
        n252 = Or(x=w457, y="Fish") -> (x .or. y?=w455:bool)
        n253 = case shown="True" w455 {
          tunnel: w458 -> [_ w461]
          tunnel: "Fish" -> [_ w459]
          frame False {
          }
          frame True {
            n254 = case shown="True" w459 {
              selector: w459 -> [w464 w465]
              tunnel: [w464 w465] -> w460
              frame False {
              }
              frame True {
                w466 = FALSE ("Tether")
                n255 = local write "Scan axis 2"(TRUE) -> ()
                n256 = local write "Tether"(w466) -> ()
                n257 = local write "Hysteresis"(w466) -> ()
                n258 = local write "Multiple tether"(w466) -> ()
                n259 = local write "Bad fit"(w466) -> ()
                n260 = local write "Good tether"(w466) -> ()
                n261 = property on="Trap D (MHz)" class="DigNum (strict)"("Val(Sgnl)"="Furthest D (MHz)") -> ()  [unwired: 2 in, 2 out]
                n262 = local read "Flow ON\nduring cal?"() -> (w467:bool)
                n263 = Or(x="Flow ON during \nfishing?", y=w467) -> (x .or. y?=w468:bool)
                n264 = Wait (ms)(milliseconds to wait=u32 500) -> ()  [unwired: 1 out]
                n265 = property on="Sample Channel\nFlow" class="Bool (strict)"("Val(Sgnl)"=w468) -> ()  [unwired: 2 in, 2 out]
              }
            }
            n266 = node-c288() -> (w463:T21)  [unwired: 4 out]
            n267 = timed-loop "Oscillate AOD" {
              timing: w463 -> [_]
              timing-out: [_] -> w462
              tunnel: w461 -> [w480]
              tunnel: w460 -> [w474]
              i -> [w482]
              stop <- w473 stop-if-true
              n268 = node-c288() -> (w481:i64)  [unwired: 1 out]
              n269 = flat-sequence {
                tunnel: w482 -> [w509]
                tunnel: w481 -> [w508]
                tunnel: w480 -> [w487]
                tunnel: w474 -> [w490]
                tunnel: [w490] -> w479
                tunnel: [w489] -> w478
                tunnel: [w486] -> w477
                tunnel: [w483] -> w475
                tunnel: w479 -> [w552]
                tunnel: w478 -> [w550]
                tunnel: w477 -> [w549]
                tunnel: [w548] -> w476
                tunnel: w475 -> [w547]
                tunnel: [w708] -> w473
                tunnel: w476 -> [w707]
                frame #0 {
                  n270 = Divide(x=w508, y=i64 1000) -> (x/y=w503:dbl)
                  n271 = Multiply(x=w503, y=w509) -> (x*y=w505:dbl)
                  n272 = local read "BD 1 Frequency 2 (MHz)"() -> (w488:dbl)
                  n273 = Multiply(x="Osc. freq. (Hz)", y=6.283185307179586) -> (x*y=w506:dbl)
                  n274 = Multiply(x=w506, y=w505) -> (x*y=w485:dbl)
                  n275 = local read "BD 1 Frequency 1 (MHz)"() -> (w493:dbl)
                  n276 = local read "BD 2 Frequency 1 (MHz)"() -> (w492:dbl)
                  n277 = case shown="True" w490 {
                    tunnel: w485 -> [w515 w520]
                    tunnel: w493 -> [_ w531]
                    tunnel: w488 -> [_ w532]
                    tunnel: [w512 w526] -> w491
                    tunnel: [FALSE w523] -> w486
                    tunnel: [0.0 w516] -> w483
                    frame False {
                      n278 = Sine(x=w515) -> (sin(x)=w513:dbl)
                      n279 = Multiply(x=w513, y="Osc. amp. (MHz)") -> (x*y=w512:dbl)
                    }
                    frame True {
                      n280 = Cosine(x=w520) -> (cos(x)=w535:dbl)
                      n281 = Subtract(x=w532, y=w531) -> (x-y=w530:dbl)
                      n282 = Decrement(x=w535) -> (x-1=w534:dbl)
                      n283 = Subtract(x=w530, y="Closest D (MHz)") -> (x-y=w527:dbl)
                      n284 = Divide(x=w534, y=-2.0) -> (x/y=w528:dbl)
                      n285 = Multiply(x=w528, y=w527) -> (x*y=w526:dbl)
                      n286 = local read "Vec Mean of T1 T2"() -> (w522:dbl[])
                      n287 = Greater?(x=w522, y="Stop F (pN)") -> (0:w524:bool[])
                      n288 = Or Array Elements(Boolean array=w524) -> (logical OR=w523:bool)
                      n289 = Divide(x=w520, y=6.283185307179586) -> (x/y=w519:dbl)
                      n290 = Round Toward +Infinity(x=w519) -> (ceil(x): smallest int >= x=w516:dbl)
                      "Attempts" <- w516
                      n291 = Greater?(x=w516, y="Attempt Limit") -> (0:w518:bool)
                      n292 = case shown="True" w518 {
                        frame False {
                        }
                        frame True {
                          n293 = local write "Fish"(FALSE ("Fish for Tether")) -> ()
                          n294 = local read "Messages"() -> (w537:string)
                          n295 = flat-sequence {
                            frame #0 {
                              n296 = call <vilib>:"Beep.vi"("use system alert? (T)"=FALSE, "duration (msec)"=u32 200, "frequency (Hz)"=u32 500) -> ()  [unwired: 9 out]
                            }
                            frame #1 {
                              n297 = Wait (ms)(milliseconds to wait=u32 100) -> ()  [unwired: 1 out]
                            }
                            frame #2 {
                              n298 = call <vilib>:"Beep.vi"("use system alert? (T)"=FALSE, "duration (msec)"=u32 200, "frequency (Hz)"=u32 500) -> ()  [unwired: 9 in]
                            }
                          }
                          n299 = call "Update messages.vi"("Message to add"="Tether fishing timeout." ("Messages"), "Old message string"=w537) -> ("New message string"=→"Messages":string)
                        }
                      }
                    }
                  }
                  n300 = Select(t=w493, s="Scan axis 2", f=w492) -> (s? t:f=w496:dbl)
                  n301 = Add(x=w491, y=w496) -> (x+y=w489:dbl)
                  n302 = Select(t=w489, s="Scan axis 2", f=w493) -> (s? t:f=w499:dbl)
                  n303 = Select(t=w492, s="Scan axis 2", f=w489) -> (s? t:f=w498:dbl)
                  n304 = local read "Y RF Frequency Limits (MHz)"() -> (w494:T16)
                  n305 = local read "X RF Frequency Limits (MHz)"() -> (w495:T16)
                  n306 = local read "BD 2 Frequency 2 (MHz)"() -> (w501:dbl)
                  n307 = local read "BD 2 Frequency 3 (MHz)"() -> (w500:dbl)
                  n308 = local read "BD 1 Frequency 3 (MHz)"() -> (w502:dbl)
                  n309 = call "set RF board frequency - interlace.vi"("Board 2 Frequency Limits"=w494, "Board 1 Frequency Limits"=w495, "FPGA VI Reference In"=w487, "Board 2 Frequency 3 (MHz)"=w500, "Board 1 Frequency 3 (MHz)"=w502, "Board 2 Frequency 2 (MHz)"=w501, "Board 2 Frequency 1 (MHz)"=w498, "Board 1 Frequency 2 (MHz)"=w488, "Board 1 Frequency 1  (MHz)"=w499) -> ()  [unwired: 1 in, 2 out]
                }
                frame #1 {
